vi "反控仪器调用.vi"(11 "设置参数":T1(ring)=enum."CODMn") -> ()   [LabVIEW 2016, in "MB SLAVE.lvlib"]
uses:
  MB SLAVE.lvlib
panel:
  in  "错误输入（无错误）":errorcluster
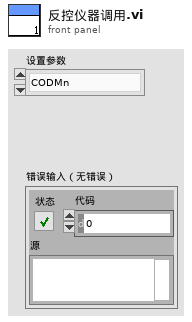
[diagram p1: front panel]
types:
  T1 = enum16{"", "CODMn", "PH", "氨氮", "总氮", "总磷", "CODCr", "电导率", "水温", "溶解氧", "浊度", "叶绿素", "藻密度", "ORP"}
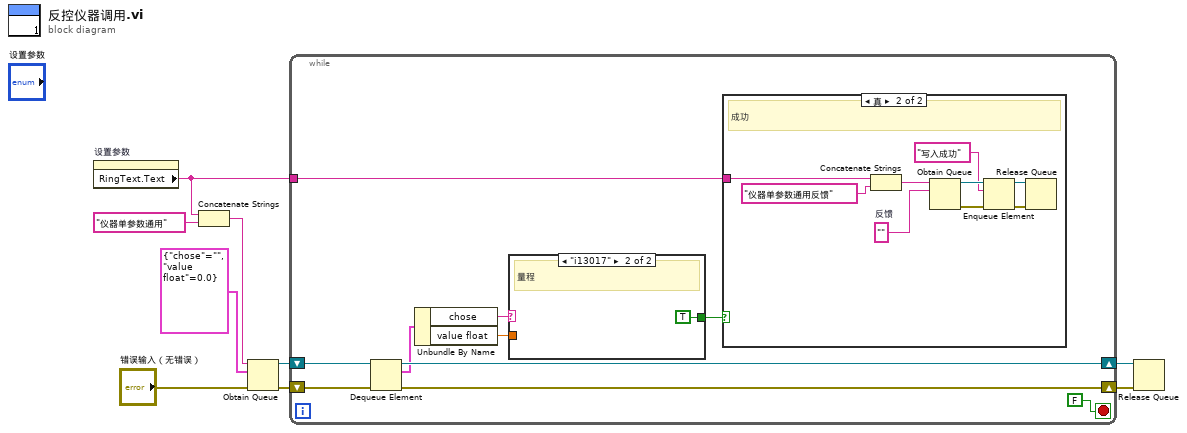
[diagram p0: block diagram]
diagram:
  n1 = property on="设置参数" class="Enum (严格)"() -> ("RingText.Text"=w1:string)  [unwired: 2 in, 2 out]
  n2 = Concatenate Strings(w1, "仪器单参数通用" ("名称（未命名）")) -> (w6:string)
  n3 = Obtain Queue(name (unnamed)=w6, element data type=cluster{"chose":string, "value float":dbl} {"chose"="", "value float"=0.0}, error in (no error)="错误输入（无错误）") -> (queue out=w5:refnum<queue>, error out=w4:errorcluster)  [unwired: 2 in, 1 out]
  n4 = while {
    shift-right: [w17] -> w3
    shift-left: w5 -> [w19]
    shift-right: [w16] -> w2
    shift-left: w4 -> [w18]
    tunnel: w1 -> [w10]
    stop <- FALSE stop-if-true
    n5 = Dequeue Element(queue=w19, error in (no error)=w18) -> (queue out=w17:refnum<queue>, element=w14:cluster{"chose":string, "value float":dbl}, error out=w16:errorcluster)  [unwired: 1 in, 1 out]
    n6 = Unbundle By Name(w14) -> ("chose"=w13:string, "value float"=w12:dbl)
    n7 = case shown="\"i13017\"" w13 {
      tunnel: w12 -> [_ _]
      tunnel: [_ TRUE] -> w11
      frame "假", Default {
      }
      frame "i13017" {
        # "量程"
      }
    }
    n8 = case shown="真" w11 {
      tunnel: w10 -> [_ w27]
      frame False {
      }
      frame True {
        w22 = ""  # 反馈
        # "成功"
        n9 = Concatenate Strings(w27, "仪器单参数通用反馈" ("名称（未命名）")) -> (w21:string)
        n10 = Obtain Queue(name (unnamed)=w21, element data type=w22) -> (queue out=w23:refnum<queue>, error out=w24:errorcluster)  [unwired: 3 in, 1 out]
        n11 = Enqueue Element(queue=w23, element="写入成功" ("元素"), error in (no error)=w24) -> (queue out=w26:refnum<queue>, error out=w25:errorcluster)  [unwired: 1 in, 1 out]
        n12 = Release Queue(queue=w26, error in (no error)=w25) -> ()  [unwired: 1 in, 3 out]
      }
    }
  }
  n13 = Release Queue(queue=w3, error in (no error)=w2) -> ()  [unwired: 1 in, 3 out]
